vi "Initialize.vi"(8 "error in":errorcluster, 10 "InstanceName":string, 11 "Chiller Cluster - 1 Channel.lvclass":refnum<class "Chiller Cluster - 1 Channel.lvclass">) -> (0 "error out":errorcluster, 3 "output cluster":refnum<class "Chiller Cluster - 1 Channel.lvclass">)   [LabVIEW 2023, in "Chiller Cluster - 1 Channel.lvclass"]
uses:
  Chiller Cluster - 1 Channel.lvclass
  Chiller Cluster - 1 Channel.lvclass/Chiller Cluster - 1 Channel.ctl
  546b7d5c-4f51-47af-9af1-567894f85656.vi
  397b3e0b-0f1b-47d9-9f6d-8a44e581e150.vi
  248f2659-eb42-462d-9a15-8e5b3aec119f.vi
  b9c13089-0281-44b9-a90f-aec73f88b65c.vi
  546b7d5c-4f51-47af-9af1-567894f85656.vi/4bc1c15b-36ab-481f-b8dd-c64075ce723a.vi
  397b3e0b-0f1b-47d9-9f6d-8a44e581e150.vi/4bc1c15b-36ab-481f-b8dd-c64075ce723a.vi
  248f2659-eb42-462d-9a15-8e5b3aec119f.vi/4bc1c15b-36ab-481f-b8dd-c64075ce723a.vi
  b9c13089-0281-44b9-a90f-aec73f88b65c.vi/4bc1c15b-36ab-481f-b8dd-c64075ce723a.vi
  <vilib>/ADAS Replay HIL/AdasHilServices/AdasHilServices Fill In Error Info Ex.vi
  Utilities/Utilities.lvlib
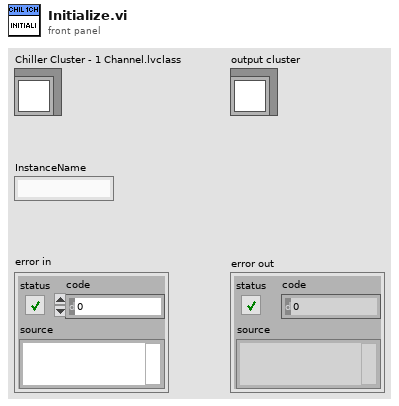
[diagram p1: front panel]
types:
  T1 = cluster{"OnOff.ACT":bool, "ErrorAcknowledge.ACT":bool}
  T2 = cluster{"OnOff.STS":i32, "Error.STS":i32, "Watchdog.STS":i32}
  T3 = cluster{"ErrorAcknowledge.ch01.ACT":bool, "OutputEnable.ch01.ACT":bool, "ControlMode.ch01.CTL":u16, "Temperature.ch01.SP":dbl, "TemperatureMIN.ch01.SP":dbl, "TemperatureMAX.ch01.SP":dbl, "TemperatureGrad.ch01.SP":dbl, "Pressure.ch01.SP":dbl, "PressureMIN.ch01.SP":dbl, "PressureMAX.ch01.SP":dbl, "PressureGrad.ch01.SP":dbl, "Flow.ch01.SP":dbl, "FlowMIN.ch01.SP":dbl, "FlowMAX.ch01.SP":dbl, "FlowGrad.ch01.SP":dbl}
  T4 = cluster{"Error.ch01.STS":i32, "OutputEnable.ch01.STS":i32, "ControlMode.ch01.STS":u16, "Temperature.ch01.AV":dbl, "Pressure.ch01.AV":dbl, "Flow.ch01.AV":dbl}
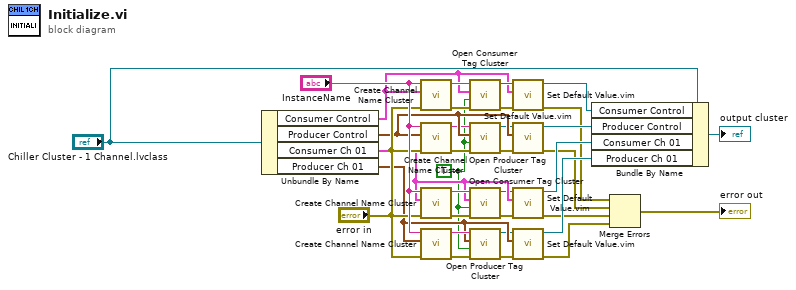
[diagram p0: block diagram]
diagram:
  w6 = TRUE ("Create if not found? (T)")
  n1 = Unbundle By Name("Chiller Cluster - 1 Channel.lvclass") -> ("Consumer Control"=w17:T1, "Producer Control"=w16:T2, "Consumer Ch 01"=w11:T3, "Producer Ch 01"=w7:T4)
  n2 = call "Create Channel Name Cluster.vi"("error in"="error in", "Cluster"=w17, "Instance Name"="InstanceName") -> ("error out"=w24:errorcluster, "Data Channel Name"=w32:string)  [unwired: 7 in]
  n3 = call "Create Channel Name Cluster.vi"("error in"="error in", "Cluster"=w16, "Instance Name"="InstanceName") -> ("error out"=w14:errorcluster, "Data Channel Name"=w15:string)  [unwired: 7 in]
  n4 = call "Create Channel Name Cluster.vi"("error in"="error in", "Cluster"=w11, "Instance Name"="InstanceName") -> ("error out"=w10:errorcluster, "Data Channel Name"=w12:string)  [unwired: 7 in]
  n5 = call "Create Channel Name Cluster.vi"("error in"="error in", "Cluster"=w7, "Instance Name"="InstanceName") -> ("error out"=w5:errorcluster, "Data Channel Name"=w8:string)  [unwired: 7 in]
  n6 = call "Open Consumer Tag Cluster.vi"("error in"=w24, "Create if not found? (T)"=w6, "Cluster"=w17, "Channel Name"=w32) -> ("error out"=w29:errorcluster, "ADAS HIL Channel"=w31:refnum<k21>)  [unwired: 6 in]
  n7 = call "Open Producer Tag Cluster.vi"("error in"=w14, "Create if not found? (T)"=w6, "Cluster"=w16, "Channel Name"=w15) -> ("error out"=w13:errorcluster, "ADAS HIL Channel"=w1:refnum<k21>)  [unwired: 6 in]
  n8 = call "Open Consumer Tag Cluster.vi"("error in"=w10, "Create if not found? (T)"=w6, "Cluster"=w11, "Channel Name"=w12) -> ("error out"=w9:errorcluster, "ADAS HIL Channel"=w2:refnum<k21>)  [unwired: 6 in]
  n9 = call "Open Producer Tag Cluster.vi"("error in"=w5, "Create if not found? (T)"=w6, "Cluster"=w7, "Channel Name"=w8) -> ("error out"=w4:errorcluster, "ADAS HIL Channel"=w3:refnum<k21>)  [unwired: 6 in]
  n10 = call "Set Default Value.vim"("error in"=w29, "Data in"=w17, "ADAS HIL Channel in"=w31) -> ("error out"=w22:errorcluster, "ADAS HIL Channel out"=w30:refnum<k21>)  [unwired: 7 in]
  n11 = call "Set Default Value.vim"("error in"=w13, "Data in"=w16, "ADAS HIL Channel in"=w1) -> ("error out"=w21:errorcluster, "ADAS HIL Channel out"=w28:refnum<k21>)  [unwired: 7 in]
  n12 = call "Set Default Value.vim"("error in"=w9, "Data in"=w11, "ADAS HIL Channel in"=w2) -> ("error out"=w20:errorcluster, "ADAS HIL Channel out"=w26:refnum<k21>)  [unwired: 7 in]
  n13 = call "Set Default Value.vim"("error in"=w4, "Data in"=w7, "ADAS HIL Channel in"=w3) -> ("error out"=w19:errorcluster, "ADAS HIL Channel out"=w25:refnum<k21>)  [unwired: 7 in]
  n14 = Bundle By Name(cluster="Chiller Cluster - 1 Channel.lvclass", "Consumer Control"=w30, "Producer Control"=w28, "Consumer Ch 01"=w26, "Producer Ch 01"=w25) -> (→"output cluster":refnum<class "Chiller Cluster - 1 Channel.lvclass">)
  n15 = Merge Errors(w22, w21, w20, w19) -> (→"error out":errorcluster)
